vi "Spreadsheet Info Dialog.vi"   [LabVIEW 2012]
panel:
  # "Excel Spreadsheet Formatting"
  # "Instructions"
  # "This VI saves the data log as a Comma Separated Value (.csv) file. CSV files can be open in Microsoft Excel, however the time formatting does not show the correct time by default. Follow the steps below to format the time correctly\n\n1. Select the Time column\n2. Click on the format dropdown \n3. Click More Number Formats...\n4. Select Custom from the Number Categories\n5. Enter hh:mm:ss.00 for custom number formatting type"
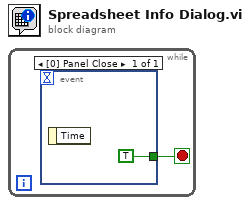
[diagram p0: block diagram]
diagram:
  n1 = while {
    stop <- w1 stop-if-true
    n2 = event shown="[0] Panel Close" {
      selector: _ -> [_]
      dyn-events: _ -> [_]
      timeout: _ -> [_]
      tunnel: [TRUE] -> w1
      event Panel Close {
        n3 = event-data() -> ()  [unwired: 1 in, 1 out]
      }
    }
  }
